vi "sub_HandleOutput.vi"(8 "error in (no error)":errorcluster, 10 "Dynamic data 2":T1, 11 "Input parameters":T2={"Measurement type"=enum."Test", "Sensor type"=enum."One channel", "Input file"="", "Output file"="test.txt", "Open after execution?"=FALSE, "Display channel"=0, "Voltage Delay (s)"=0.5, "Switch Delay (s)"=0.01, "VISA resource name source"="", "VISA resource name LCR"="", "Voltage Limit (V)"=1000.0, "Enable Voltage Auto Range (T:Enable)"=TRUE, "Voltage Manual Range (1.0)"=1.0, "Compliance  Level (uA)"=10.0} {"Voltage Limit (V)" format="%#_13g"; "Voltage Delay (s)" format="%#_13g"; "Switch Delay (s)" format="%#_13g"}) -> (0 "error out":errorcluster, 2 "Dynamic data":T1, 3 "Input parameters":T2={"Measurement type"=enum."Test", "Sensor type"=enum."One channel", "Input file"="", "Output file"="test.txt", "Open after execution?"=FALSE, "Display channel"=0, "Voltage Delay (s)"=0.5, "Switch Delay (s)"=0.01, "VISA resource name source"="", "VISA resource name LCR"="", "Voltage Limit (V)"=1000.0, "Enable Voltage Auto Range (T:Enable)"=TRUE, "Voltage Manual Range (1.0)"=1.0, "Compliance  Level (uA)"=10.0} {"Voltage Limit (V)" format="%#_13g"; "Voltage Delay (s)" format="%#_13g"; "Switch Delay (s)" format="%#_13g"})   [LabVIEW 2015]
uses:
  <vilib>/Utility/file.llb/Write Delimited Spreadsheet (string).vi
  Input_parameters.ctl
  Dynamic_data.ctl
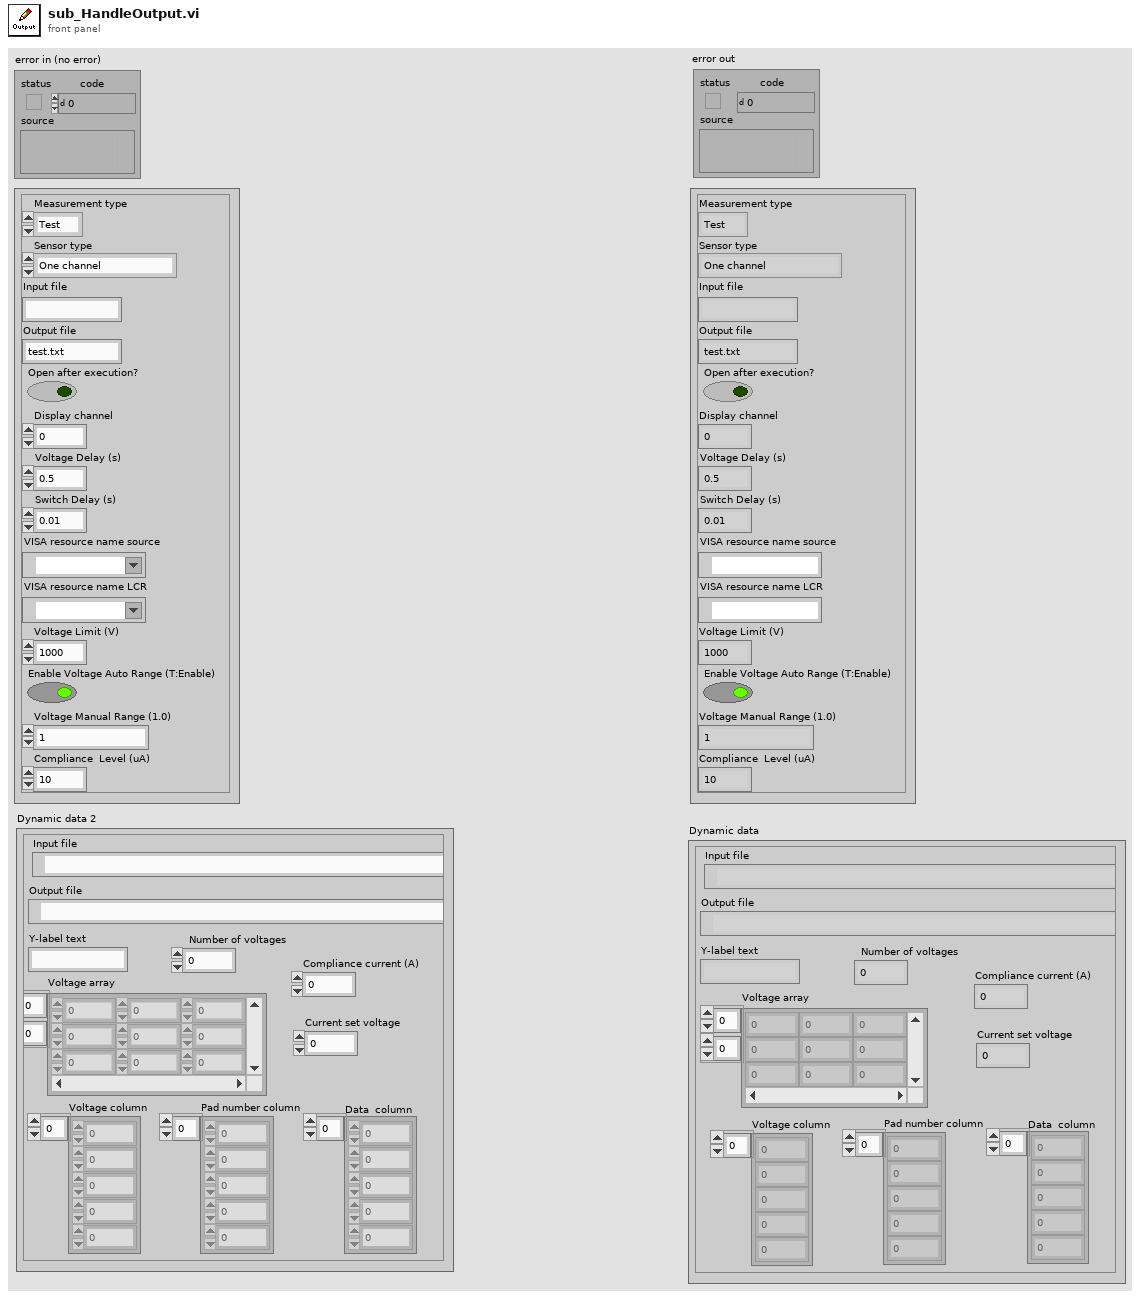
[diagram p1: front panel]
types:
  T1 = typedef "Dynamic_data.ctl" = cluster{"Input file":path, "Output file":path, "Y-label text":string, "Voltage array":dbl[][], "Current set voltage":dbl, "Voltage column":dbl[], "Pad number column":dbl[], "Data  column":dbl[], "Number of voltages":i32, "Compliance current (A)":dbl}
  T2 = typedef "Input_parameters.ctl" = cluster{"Measurement type":enum16{"IV", "CV", "Test"}, "Sensor type":enum16{"6''", "8''", "One channel"}, "Input file":string, "Output file":string, "Open after execution?":bool, "Display channel":i32, "Voltage Delay (s)":dbl, "Switch Delay (s)":dbl, "VISA resource name source":refnum<visa-resource-name>, "VISA resource name LCR":refnum<visa-resource-name>, "Voltage Limit (V)":dbl, "Enable Voltage Auto Range (T:Enable)":bool, "Voltage Manual Range (1.0)":dbl, "Compliance  Level (uA)":dbl}
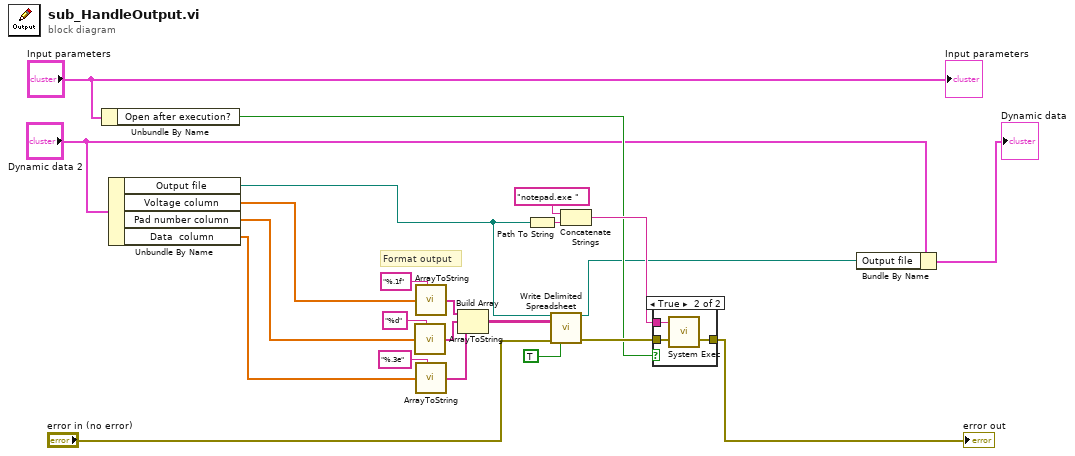
[diagram p0: block diagram]
diagram:
  # "Format output"
  n1 = Unbundle By Name("Input parameters") -> ("Open after execution?"=w8:bool)
  n2 = Unbundle By Name("Dynamic data 2") -> ("Output file"=w4:path, "Voltage column"=w3:dbl[], "Pad number column"=w2:dbl[], "Data  column"=w1:dbl[])
  n3 = call "ArrayToString.vi"("Format"="%d", "Input 1D array"=w2) -> ("Output 1D array"=w17:string[])  [unwired: 7 in]
  n4 = call "ArrayToString.vi"("Format"="%.1f", "Input 1D array"=w3) -> ("Output 1D array"=w18:string[])  [unwired: 7 in]
  n5 = call "ArrayToString.vi"("Format"="%.3e", "Input 1D array"=w1) -> ("Output 1D array"=w19:string[])  [unwired: 7 in]
  n6 = Build Array(w18, w17, w19) -> (w16:string[][])
  n7 = Path To String(path=w4) -> (string=w15:string)
  n8 = call-poly <vilib>:"Write Delimited Spreadsheet.vi"("file path (dialog if empty)"=w4, "2D data"=w16, "error in (no error)"="error in (no error)", "transpose? (no:F)"=TRUE) -> ("new file path (Not A Path if cancelled)"=w7:path, "error out"=w12:errorcluster)  [unwired: 10 in]
  n9 = Concatenate Strings("notepad.exe " ("string"), w15) -> (w13:string)
  n10 = case shown="True" w8 {
    tunnel: w13 -> [_ w27]
    tunnel: w12 -> [w24 w26]
    tunnel: [w24 w25] -> w9
    frame False {
    }
    frame True {
      n11 = call <vilib>:"System Exec.vi"("error in (no error)"=w26, "command line"=w27) -> ("error out"=w25:errorcluster)  [unwired: 6 in, 3 out]
    }
  }
  "error out" <- w9
  n12 = Bundle By Name(cluster="Dynamic data 2", "Output file"=w7) -> (→"Dynamic data":T1)
  "Input parameters" <- "Input parameters"
